vi "FormatBounceData(LC).vi"() -> ()   [LabVIEW 2018]
uses:
  <vilib>/Utility/file.llb/Read Delimited Spreadsheet (string).vi
  <vilib>/Utility/file.llb/Write Delimited Spreadsheet (DBL).vi
  <vilib>/Utility/file.llb/Write Delimited Spreadsheet (string).vi
panel:
  out "cancelled":bool
  out "out folder":path caption="selected path"
  in  "Use File Dialog(T)":bool
  in  "WriteFile(T)":bool
  out "origfile":string
  out "done_filename":string
  out "name":string
  out "done file":path
  out "data_out":string[][](array[string])
  out "data_header_out":string[](array[string])=["SER NUM", "AMPL (DB)", "FREQ (MHZ)", "ANT", "TX ANT", "RX ANT"]
  out "FileHeader":string[][](array[string])
  out "Chan_header":string[](array[string])
  out "Chan_Data":string[][](array[string])
  out "dut_sn":string
  out "DutSnIndex":i32
  out "freq_data":string[](array[string])
  out "ampl_data":string[](array[string])
  out "AmplLen":i32
  out "FreqStartIndex":i32
  out "FreqStopIndex":i32
  out "AmplStopIndex":i32
  out "AmplStartIndex":i32
  out "subarray":string[](array[string])
  out "origpath":string
  out "size":i32
  out "DataRowIndex":i32
  out "HeaderRowIndex":i32
  out "all rows":string[][](array[string])
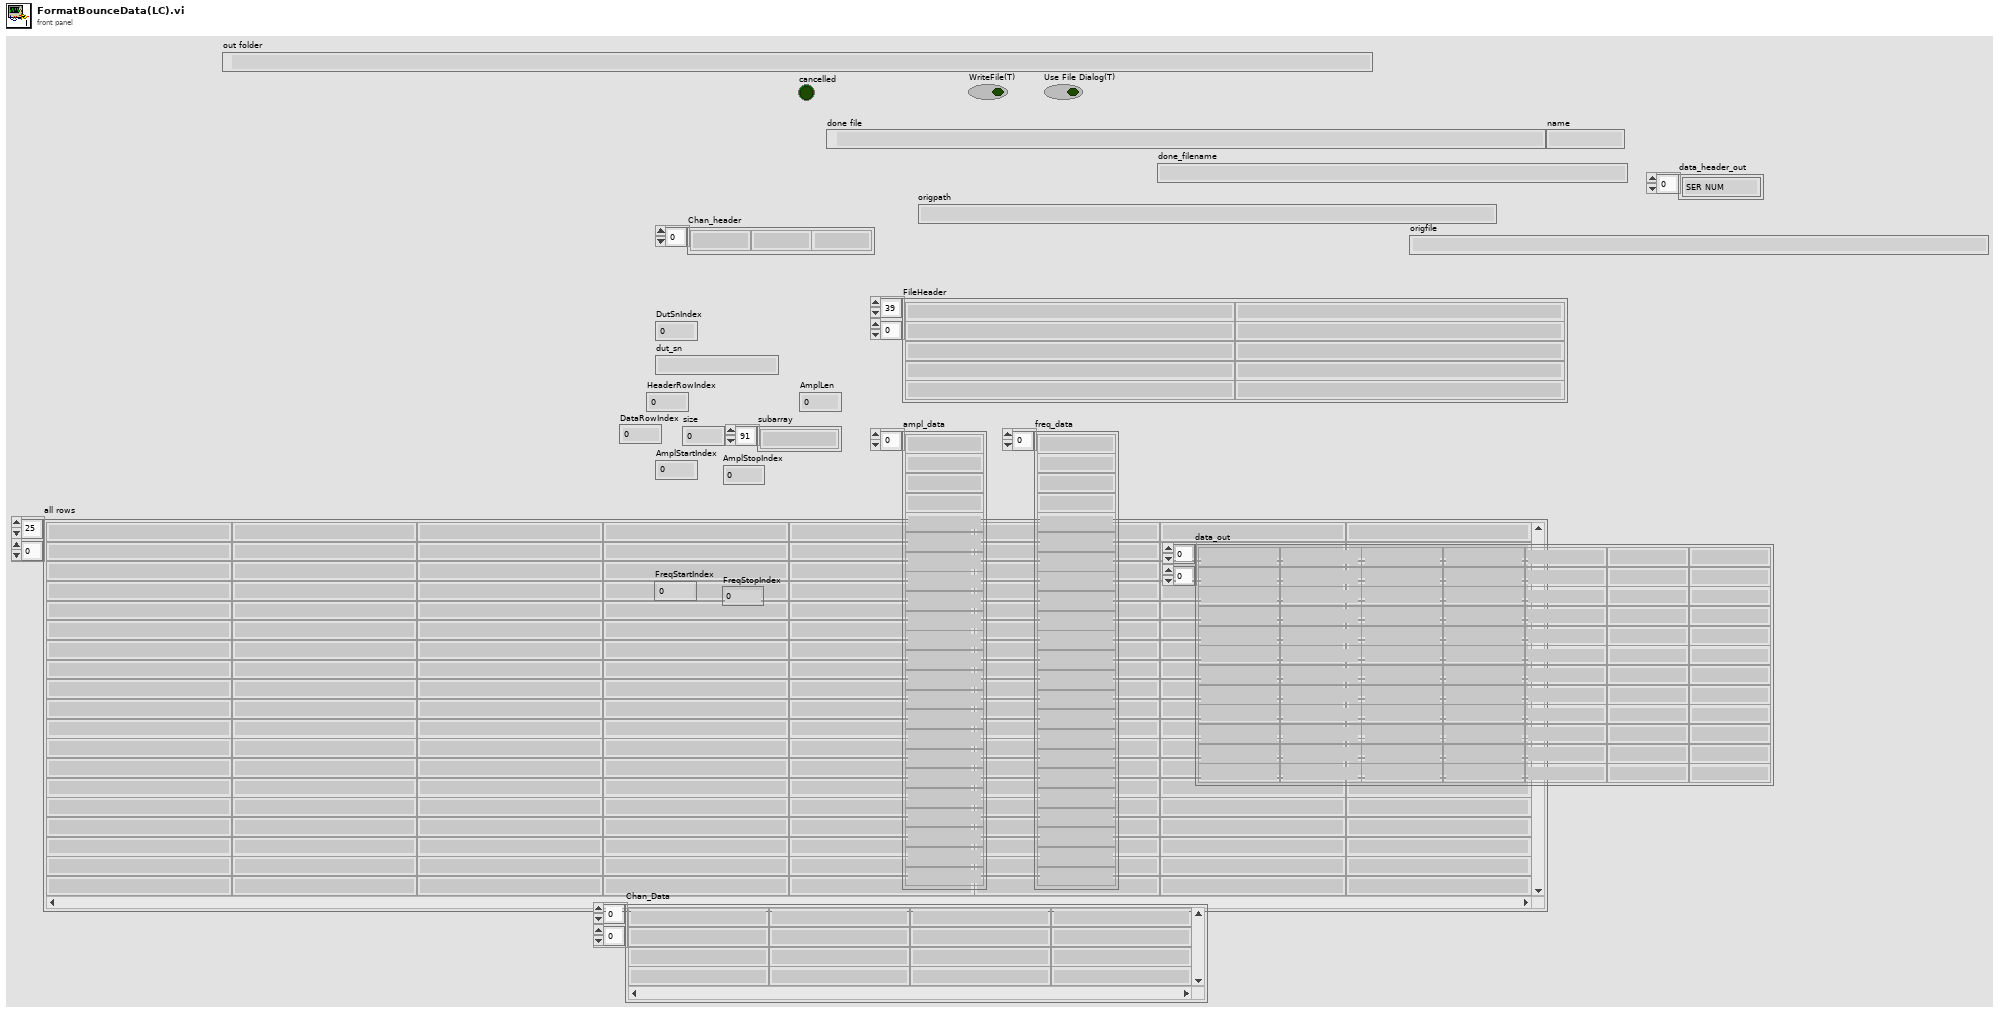
[diagram p1: front panel]
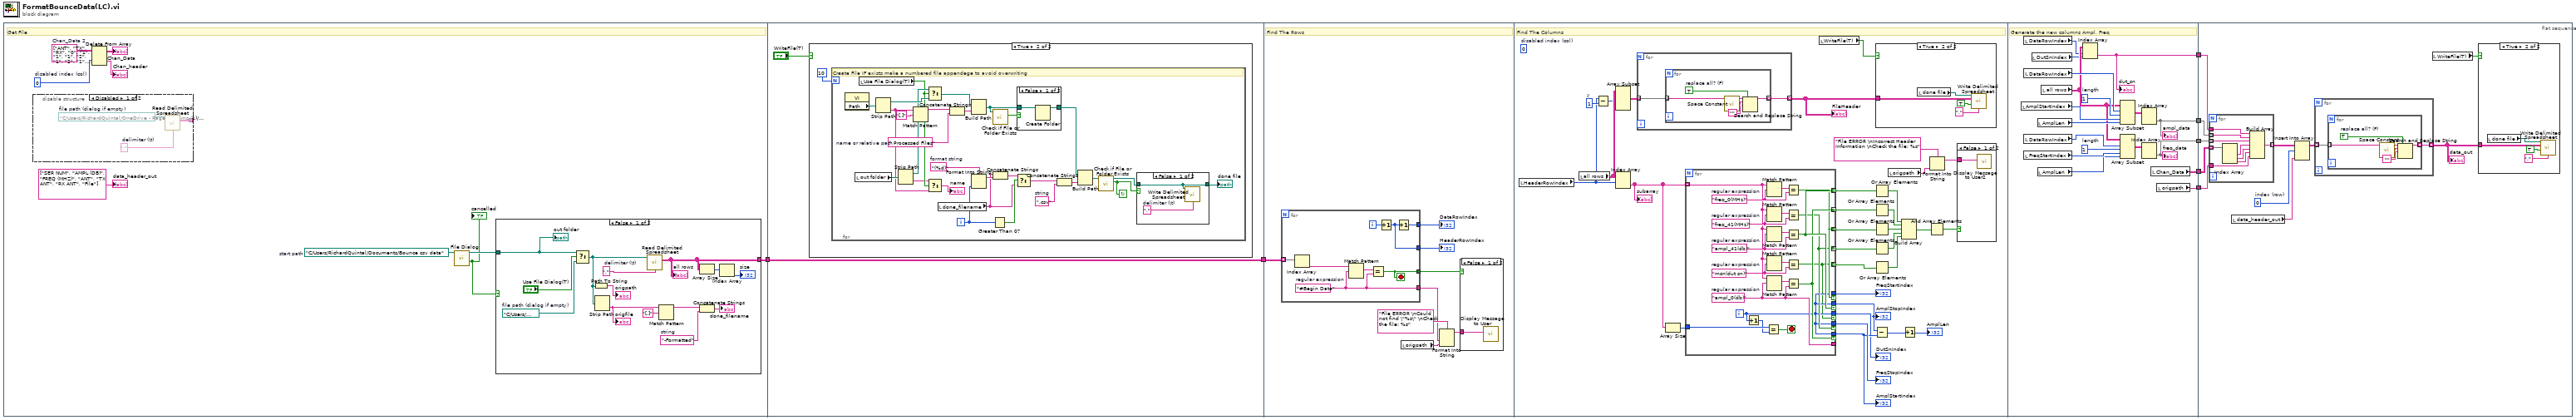
[diagram p0: block diagram]
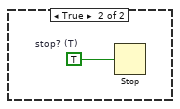
[diagram p2: hidden frame]
diagram:
  n1 = flat-sequence {
    tunnel: [w16] -> w2
    tunnel: w2 -> [w36]
    tunnel: [w36] -> w1
    tunnel: w1 -> [w80]
    tunnel: [w157] -> w7
    tunnel: [w156] -> w6
    tunnel: [w155] -> w5
    tunnel: [w154] -> w4
    tunnel: [w153] -> w3
    tunnel: w7 -> [w181]
    tunnel: w6 -> [w180]
    tunnel: w5 -> [w179]
    tunnel: w4 -> [w178]
    tunnel: w3 -> [w174]
    frame #0 {
      w9 = path "C:/Users/RichardQuintal/Documents/Bounce csv data"  # start path
      w12 = 0  # disabled index (col)
      w15 = string[][] [["ANT", "TX", "RX"], ["0", "1", "1"], ["1", "2", "1"], ["2", "1", "2"], ["3", "3", "1"], ["4", "2", "2"], ["5", "4", "1"], ["6", "3", "2"], ["7", "2", "3"], ["8", "4", "2"], ["9", "3", "3"], ["10", "5", "2"], ["11", "4", "3"], ["12", "3", "4"], ["13", "5", "3"], ["14", "4", "4"], ["15", "6", "3"], ["16", "5", "4"], ["17", "7", "3"], ["18", "6", "4"], ["19", "5", "5"], ["20", "7", "4"], ["21", "6", "5"], ["22", "8", "4"], ["23", "7", "5"], ["24", "6", "6"], ["25", "8", "5"], ["26", "7", "6"], ["27", "9", "5"], ["28", "8", "6"], ["29", "10", "5"], ["30", "9", "6"], ["31", "8", "7"], ["32", "10", "6"], ["33", "9", "7"], ["34", "11", "6"], ["35", "10", "7"], ["36", "9", "8"], ["37", "11", "7"], ["38", "10", "8"], ["39", "12", "7"], ["40", "11", "8"], ["41", "12", "8"]]  # Chan_Data 2
      # "Get File"
      n2 = disable-structure shown="Disabled" {
        disable-tunnel: [w33 _] -> _
        frame Disabled {
          w32 = ","  # delimiter (\t)
          w34 = path "C:/Users/RichardQuintal/OneDrive - Rage Systems (1)/Documents - Rage Test Lab/Software/Labview Snips/Ricks Vis/LeidosMastMap2.csv"  # file path (dialog if empty)
          n3 = call-poly <vilib>:"Read Delimited Spreadsheet.vi"("file path (dialog if empty)"=w34, "delimiter (\\t)"=w32) -> ("all rows"=w33:string[][])  [unwired: 8 in, 5 out]
        }
        frame Enabled {
        }
      }
      n4 = Delete From Array(array=w15, index (row)=w12) -> (deleted portion=→"Chan_header":string[], array with subset deleted=→"Chan_Data":string[][])  [unwired: 2 in]
      n5 = call "File Dialog"("start path"=w9) -> ("selected path"=w10:path, "cancelled"=w8:bool)  [unwired: 11 in, 2 out]
      "cancelled" <- w8
      n6 = case shown="False" w8 {
        tunnel: [w29 _] -> w16
        tunnel: w10 -> [w18 _]
        frame False {
          w23 = "-Formatted"  # string
          w30 = ","  # delimiter (\t)
          w19 = path "C:/Users/RichardQuintal/Desktop/WAM-LC_BOUNCE_SN_RA26030002-RTP2_ 2603_04072026120455.csv"  # file path (dialog if empty)
          n7 = Select(t=w18, s="Use File Dialog(T)", f=w19) -> (s? t:f=w20:path)
          n8 = Path To String(path=w20) -> (string=→"origpath":string)
          n9 = Strip Path(path=w20) -> (name=w21:string)  [unwired: 1 out]
          "origfile" <- w21
          n10 = call-poly <vilib>:"Read Delimited Spreadsheet.vi"("file path (dialog if empty)"=w20, "delimiter (\\t)"=w30) -> ("all rows"=w29:string[][])  [unwired: 8 in, 5 out]
          "all rows" <- w29
          n11 = Match Pattern(string=w21, regular expression="[.]") -> (before substring=w25:string)  [unwired: 1 in, 3 out]
          n12 = Array Size(array=w29) -> (size(s)=w28:i32[])
          n13 = Concatenate Strings(w25, w23) -> (→"done_filename":string)
          n14 = Index Array(array=w28) -> (element=→"size":i32)  [unwired: 1 in]
          "out folder" <- w18
        }
        frame True {
          w31 = TRUE  # stop? (T)
          n15 = Stop(stop? (T)=w31) -> ()
        }
      }
      "data_header_out" <- string[] ["SER NUM", "AMPL (DB)", "FREQ (MHZ)", "ANT", "TX ANT", "RX ANT", "File"]
    }
    frame #1 {
      n16 = case shown="True" "WriteFile(T)" {
        frame False {
        }
        frame True {
          n17 = for {
            N: 10 -> [_]
            i -> [w51]
            stop <- w47 continue-if-true
            w53 = ".csv"  # string
            w57 = "(%d)"  # format string
            w60 = " Processed Files"  # name or relative path
            # "Create File IF exists make a numbered file appendege to avoid overwriting"
            n18 = property class="VI"() -> ("Path"=w62:path)  [unwired: 2 in, 2 out]
            n19 = local read "out folder"() -> (w42:path)
            n20 = local read "Use File Dialog(T)"() -> (w41:bool)
            n21 = Strip Path(path=w62) -> (stripped path=w45:path, name=w40:string)
            n22 = Strip Path(path=w42) -> (stripped path=w43:path, name=w38:string)
            n23 = Match Pattern(string=w40, regular expression="[.]") -> (before substring=w65:string)  [unwired: 1 in, 3 out]
            n24 = Select(t=w43, s=w41, f=w45) -> (s? t:f=w44:path)
            n25 = Select(t=w38, s=w41, f=w40) -> (s? t:f=→"name":string)
            n26 = local read "done_filename"() -> (w49:string)
            n27 = Concatenate Strings(w65, w60) -> (w64:string)
            n28 = Build Path(base path=w44, name or relative path=w64) -> (appended path=w66:path)
            n29 = Format Into String(format string=w57, w51) -> (resulting string=w52:string)  [unwired: 2 in, 1 out]
            n30 = Greater Than 0?(x=w51) -> (x > 0?=w50:bool)
            n31 = call <vilib>:"Check if File or Folder Exists.vi"("path"=w66) -> ("file or folder exists?"=w63:bool)  [unwired: 8 in, 2 out]
            n32 = Concatenate Strings(w49, w52) -> (w56:string)
            n33 = Select(t=w56, s=w50, f=w49) -> (s? t:f=w55:string)
            n34 = case shown="False" w63 {
              tunnel: w66 -> [w71 w72]
              tunnel: [w70 w72] -> w59
              frame False {
                n35 = Create Folder(path (use dialog)=w71) -> (created path=w70:path)  [unwired: 2 in, 2 out]
              }
              frame True {
              }
            }
            n36 = Concatenate Strings(w55, w53) -> (w54:string)
            n37 = Build Path(base path=w59, name or relative path=w54) -> (appended path=w58:path)
            n38 = call <vilib>:"Check if File or Folder Exists.vi"("path"=w58) -> ("file or folder exists?"=w47:bool, "dup path"=w48:path)  [unwired: 8 in, 1 out]
            n39 = case shown="False" w47 {
              tunnel: w48 -> [w67 w69]
              tunnel: [w67 w69] -> w46
              frame False {
                w68 = ","  # delimiter (\t)
                n40 = call-poly <vilib>:"Write Delimited Spreadsheet.vi"("file path (dialog if empty)"=w67, "delimiter (\\t)"=w68) -> ()  [unwired: 12 in, 2 out]
              }
              frame True {
              }
            }
            "done file" <- w46
          }
        }
      }
    }
    frame #2 {
      # "Find The Rows"
      n41 = for {
        tunnel: w80 -> [w89] mode=indexing
        tunnel: [w85] -> w76
        tunnel: [w84] -> w79
        tunnel: [w83] -> w78
        tunnel: [w82] -> w74
        i -> [w86]
        stop <- w85 stop-if-true
        w82 = "#Begin Data"  # regular expression
        n42 = Index Array(array=w89) -> (element=w88:string)  [unwired: 1 in]
        n43 = Match Pattern(string=w88, regular expression=w82) -> (match substring=w87:string)  [unwired: 1 in, 3 out]
        n44 = Equal?(x=w87, y=w82) -> (x = y?=w85:bool)
        n45 = Increment(x=w86) -> (x+1=w84:i32)
        n46 = Increment(x=w84) -> (x+1=w83:i32)
      }
      "HeaderRowIndex" <- w79
      "DataRowIndex" <- w78
      n47 = local read "origpath"() -> (w73:string)
      n48 = Format Into String(format string="File ERROR \nCould not find \"%s\" \nCheck the file: %s", w74, w73) -> (resulting string=w75:string)  [unwired: 2 in, 1 out]
      n49 = case shown="False" w76 {
        tunnel: w75 -> [w81 _]
        frame False {
          n50 = call "Display Message to User"("Message"=w81) -> ()  [unwired: 9 in, 2 out]
        }
        frame True {
        }
      }
    }
    frame #3 {
      w94 = 1  # y
      (unwired) 0  # disabled index (col)
      # "Find The Columns"
      n51 = local read "HeaderRowIndex"() -> (w93:i32)
      n52 = local read "all rows"() -> (w95:string[][])
      n53 = Subtract(x=w93, y=w94) -> (x-y=w92:i32)
      n54 = Array Subset(array=w95, length (row)=w92) -> (w91:string[][])  [unwired: 3 in]
      n55 = Index Array(array=w95, index (row)=w93) -> (element=w120:string[])  [unwired: 1 in]
      "subarray" <- w120
      n56 = for {
        tunnel: w91 -> [w122] mode=indexing
        tunnel: [w121] -> w90 mode=indexing
        n57 = for {
          tunnel: w122 -> [w125] mode=indexing
          tunnel: [w123] -> w121 mode=indexing
          w124 = TRUE  # replace all? (F)
          n58 = call <vilib>:"Space Constant.vi"() -> ("String"=w127:string)
          n59 = Search and Replace String(replace all?=w124, input string=w125, search string=w127, replace string="") -> (result string=w123:string)  [unwired: 4 in, 3 out]
        }
      }
      "FileHeader" <- w90
      n60 = Array Size(array=w120) -> (size(s)=w119:i32)
      n61 = for {
        tunnel: w120 -> [w137] mode=indexing
        tunnel: [w151] -> _
        tunnel: [w134] -> w102 if=w140
        tunnel: [w134] -> w103 if=w141
        tunnel: w119 -> [w148]
        tunnel: [w134] -> w118 if=w139
        tunnel: [w134] -> w117 if=w138
        tunnel: [w141] -> w113 mode=indexing
        tunnel: [w140] -> w112 mode=indexing
        tunnel: [w139] -> w111 mode=indexing
        tunnel: [w138] -> w110 mode=indexing
        tunnel: [w134] -> w99 if=w133
        tunnel: [w133] -> w98 mode=indexing
        i -> [w134]
        stop <- w147 stop-if-true
        w135 = "msn(dut sn)"  # regular expression
        w143 = "freq_41(MHz)"  # regular expression
        w144 = "freq_0(MHz)"  # regular expression
        w150 = "ampl_41(db)"  # regular expression
        w151 = "ampl_0(db)"  # regular expression
        n62 = Increment(x=w134) -> (x+1=w146:i32)
        n63 = Equal?(x=w148, y=w146) -> (x = y?=w147:bool)
        n64 = Match Pattern(string=w137, regular expression=w144) -> (match substring=w145:string)  [unwired: 1 in, 3 out]
        n65 = Match Pattern(string=w137, regular expression=w143) -> (match substring=w142:string)  [unwired: 1 in, 3 out]
        n66 = Match Pattern(string=w137, regular expression=w150) -> (match substring=w149:string)  [unwired: 1 in, 3 out]
        n67 = Match Pattern(string=w137, regular expression=w135) -> (match substring=w136:string)  [unwired: 1 in, 3 out]
        n68 = Match Pattern(string=w137, regular expression=w151) -> (match substring=w152:string)  [unwired: 1 in, 3 out]
        n69 = Equal?(x=w145, y=w144) -> (x = y?=w139:bool)
        n70 = Equal?(x=w142, y=w143) -> (x = y?=w138:bool)
        n71 = Equal?(x=w149, y=w150) -> (x = y?=w141:bool)
        n72 = Equal?(x=w136, y=w135) -> (x = y?=w133:bool)
        n73 = Equal?(x=w152, y=w151) -> (x = y?=w140:bool)
      }
      "AmplStartIndex" <- w102
      "AmplStopIndex" <- w103
      "FreqStartIndex" <- w118
      "FreqStopIndex" <- w117
      "DutSnIndex" <- w99
      n74 = local read "WriteFile(T)"() -> (w96:bool)
      n75 = Subtract(x=w103, y=w102) -> (x-y=w101:i32)
      n76 = Or Array Elements(Boolean array=w113) -> (logical OR=w109:bool)
      n77 = Or Array Elements(Boolean array=w112) -> (logical OR=w108:bool)
      n78 = Or Array Elements(Boolean array=w111) -> (logical OR=w107:bool)
      n79 = Or Array Elements(Boolean array=w110) -> (logical OR=w106:bool)
      n80 = Or Array Elements(Boolean array=w98) -> (logical OR=w97:bool)
      n81 = case shown="True" w96 {
        tunnel: w90 -> [_ w128]
        frame False {
        }
        frame True {
          n82 = local read "done file"() -> (w131:path)
          n83 = call-poly <vilib>:"Write Delimited Spreadsheet.vi"("file path (dialog if empty)"=w131, "2D data"=w128, "append to file? (new file:F)"=TRUE, "delimiter (\\t)"="," ("delimiter (\\t)")) -> ()  [unwired: 10 in, 2 out]
        }
      }
      n84 = local read "origpath"() -> (w114:string)
      n85 = Build Array(w109, w108, w107, w106, w97) -> (w105:bool[])
      n86 = Increment(x=w101) -> (x+1=→"AmplLen":i32)
      n87 = And Array Elements(Boolean array=w105) -> (logical AND=w104:bool)
      n88 = Format Into String(format string="File ERROR \nIncorrect Header Information \nCheck the file: %s", w114) -> (resulting string=w116:string)  [unwired: 2 in, 1 out]
      n89 = case shown="False" w104 {
        tunnel: w116 -> [w132 _]
        frame False {
          n90 = call "Display Message to User2"("Message"=w132) -> ()  [unwired: 9 in, 2 out]
        }
        frame True {
        }
      }
    }
    frame #4 {
      w162 = 1  # length
      w167 = 1  # length
      # "Generate the new columns Ampl, Freq"
      n91 = local read "AmplStartIndex"() -> (w169:i32)
      n92 = local read "DataRowIndex"() -> (w159:i32)
      n93 = local read "DataRowIndex"() -> (w170:i32)
      n94 = local read "DataRowIndex"() -> (w165:i32)
      n95 = local read "FreqStartIndex"() -> (w164:i32)
      n96 = local read "DutSnIndex"() -> (w158:i32)
      n97 = local read "AmplLen"() -> (w168:i32)
      n98 = local read "AmplLen"() -> (w163:i32)
      n99 = local read "all rows"() -> (w160:string[][])
      n100 = Index Array(array=w160, index (row)=w159, index (col)=w158) -> (element=w157:string)
      "dut_sn" <- w157
      n101 = Array Subset(array=w160, index (row)=w170, length (row)=w167, index (col)=w169, length (col)=w168) -> (w166:string[][])
      n102 = Array Subset(array=w160, index (row)=w165, length (row)=w162, index (col)=w164, length (col)=w163) -> (w161:string[][])
      n103 = Index Array(array=w166) -> (element=w155:string[])  [unwired: 2 in]
      "ampl_data" <- w155
      n104 = Index Array(array=w161) -> (element=w156:string[])  [unwired: 2 in]
      "freq_data" <- w156
      n105 = local read "Chan_Data"() -> (w154:string[][])
      n106 = local read "origpath"() -> (w153:string)
    }
    frame #5 {
      w175 = 0  # index (row)
      n107 = for {
        tunnel: w181 -> [w200]
        tunnel: w180 -> [w195] mode=indexing
        tunnel: w179 -> [w194] mode=indexing
        tunnel: w178 -> [w201] mode=indexing
        tunnel: [w196] -> w177 mode=indexing
        tunnel: w174 -> [w193]
        n108 = Index Array(array=w201) -> (element #1=w199:string, element #2=w198:string, element #3=w197:string)  [unwired: 3 in]
        n109 = Build Array(w200, w194, w195, w199, w198, w197, w193) -> (w196:string[])
      }
      n110 = local read "data_header_out"() -> (w176:string[])
      n111 = Insert Into Array(array=w177, index (row)=w175, new element=w176) -> (w172:string[][])  [unwired: 1 in]
      n112 = for {
        tunnel: w172 -> [w183] mode=indexing
        tunnel: [w182] -> w171 mode=indexing
        n113 = for {
          tunnel: w183 -> [w187] mode=indexing
          tunnel: [w185] -> w182 mode=indexing
          w184 = TRUE  # replace all? (F)
          n114 = call <vilib>:"Space Constant.vi"() -> ("String"=w188:string)
          n115 = Search and Replace String(replace all?=w184, input string=w187, search string=w188, replace string="") -> (result string=w185:string)  [unwired: 4 in, 3 out]
        }
      }
      "data_out" <- w171
      n116 = local read "WriteFile(T)"() -> (w173:bool)
      n117 = case shown="True" w173 {
        tunnel: w171 -> [_ w189]
        frame False {
        }
        frame True {
          n118 = local read "done file"() -> (w192:path)
          n119 = call-poly <vilib>:"Write Delimited Spreadsheet.vi"("file path (dialog if empty)"=w192, "2D data"=w189, "append to file? (new file:F)"=TRUE, "delimiter (\\t)"="," ("delimiter (\\t)")) -> ()  [unwired: 10 in, 2 out]
        }
      }
    }
  }
